vi "Message_Handler_Data.vi"(7 "Action":T5, 8 "error in (no error)":errorcluster, 9 "Time_Out":i32, 11 "Message_IN":T1={"Message Command"=enum."Process_Photo", "Parametr"={"Frame"=refnum, "Time Stamp"=timestamp(0 s since 1904-01-01), "#Frame"=0}}) -> (0 "error out":errorcluster, 1 "timed out?":bool, 3 "Message_OUT":T1={"Message Command"=enum."Process_Photo", "Parametr"={"Frame"=refnum, "Time Stamp"=timestamp(0 s since 1904-01-01), "#Frame"=0}})   [LabVIEW 2024, in "Data_Procesing.lvlib" / "Message_Handler_Data.lvlib"]
uses:
  Message_Handler_Data.lvlib
  typedeff_CommunicationModuleAction_Data.ctl
  typedeff_Message_Data.ctl
  typedeff_Message_Command_Data.ctl
  typedeff_Message_Parameters_Data.ctl
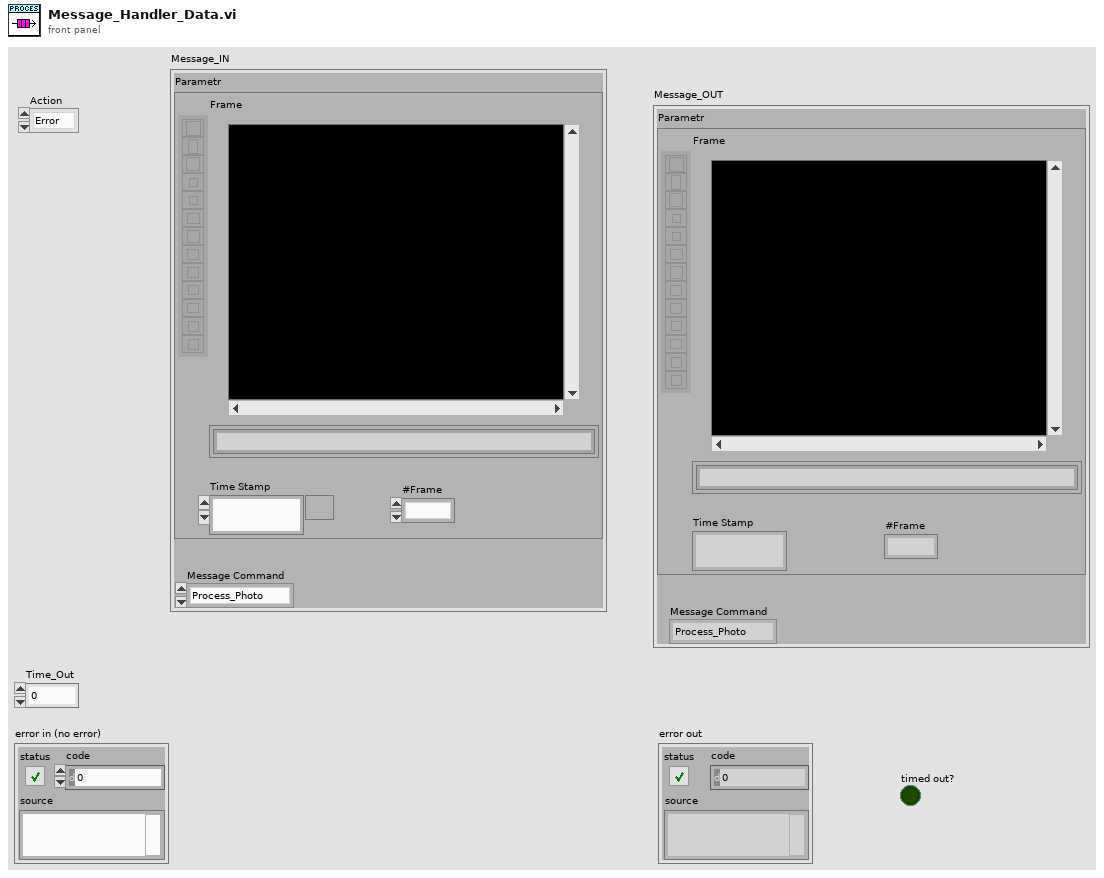
[diagram p1: front panel]
types:
  T1 = typedef "Data_Procesing.lvlib/Message_Handler_Data.lvlib/typedeff_Message_Data.ctl" = cluster{"Message Command":T2, "Parametr":T3}
  T2 = typedef "Data_Procesing.lvlib/Message_Handler_Data.lvlib/typedeff_Message_Command_Data.ctl" = enum16{"No MEssage", "Process_Photo"}
  T3 = typedef "Data_Procesing.lvlib/Message_Handler_Data.lvlib/typedeff_Message_Parameters_Data.ctl" = cluster{"Frame":T4, "Time Stamp":timestamp, "#Frame":u32}
  T4 = typedef "IMAQ Image.ctl" = refnum<image>
  T5 = typedef "Data_Procesing.lvlib/Message_Handler_Data.lvlib/typedeff_CommunicationModuleAction_Data.ctl" = enum16{"Error", "Init", "Send Msg", "Recive Msg", "Shut Down"}
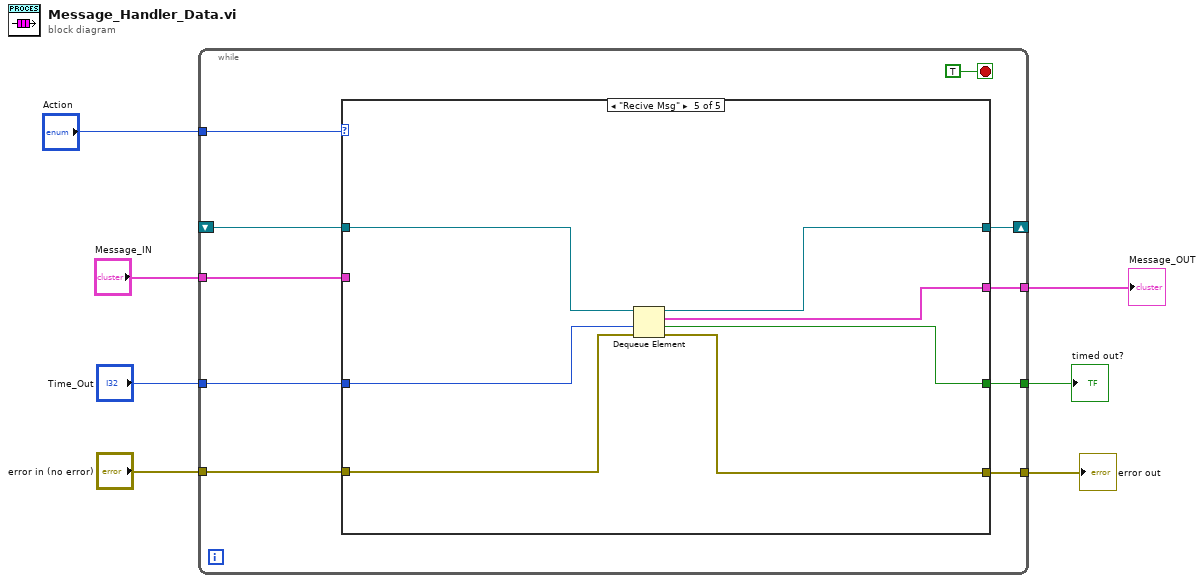
[diagram p0: block diagram]
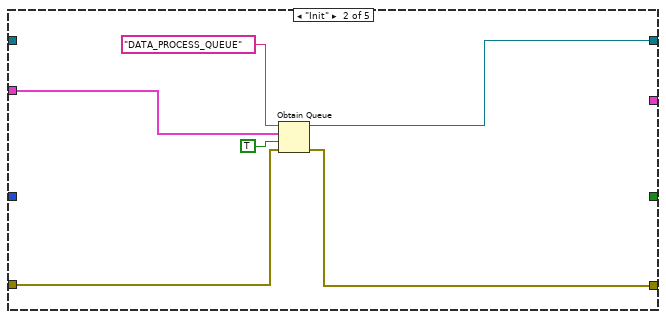
[diagram p3: hidden frame]
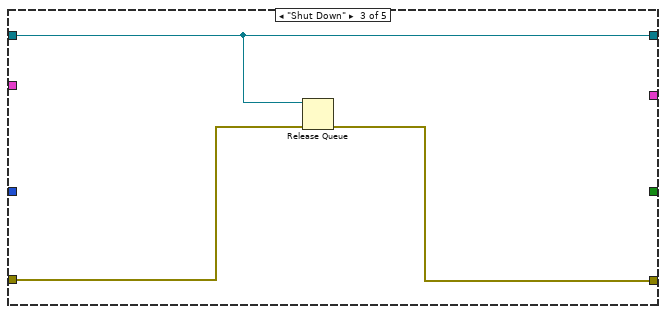
[diagram p4: hidden frame]
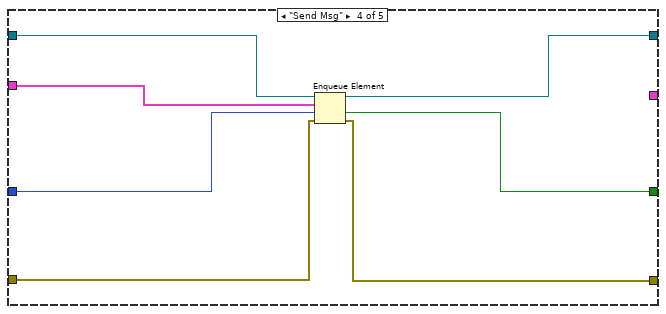
[diagram p5: hidden frame]
diagram:
  n1 = while {
    tunnel: "Action" -> [w16]
    tunnel: "error in (no error)" -> [w15]
    shift-right: [w14] -> _
    shift-left: _ -> [w13]
    tunnel: [w12] -> w6
    tunnel: "Time_Out" -> [w11]
    tunnel: [w10] -> w2
    tunnel: "Message_IN" -> [w9]
    tunnel: [w8] -> w4
    stop <- TRUE stop-if-true
    n2 = case shown="\"Recive Msg\"" w16 {
      tunnel: w15 -> [_ w23 w27 w31 w36]
      tunnel: [w18 w22 w25 w32 w39] -> w14
      tunnel: w13 -> [w18 _ w25 w34 w41]
      tunnel: [_ w21 w26 w30 w37] -> w12
      tunnel: w11 -> [_ _ _ w33 w40]
      tunnel: [_ _ _ _ w38] -> w10
      tunnel: w9 -> [_ w19 _ w29 _]
      tunnel: [_ _ _ w28 w35] -> w8
      frame "Error", Default {
      }
      frame "Init" {
        n3 = Obtain Queue(name (unnamed)="DATA_PROCESS_QUEUE", element data type=w19, create if not found? (T)=TRUE, error in (no error)=w23) -> (queue out=w22:refnum<queue>, error out=w21:errorcluster)  [unwired: 1 in, 1 out]
      }
      frame "Shut Down" {
        n4 = Release Queue(queue=w25, error in (no error)=w27) -> (error out=w26:errorcluster)  [unwired: 1 in, 2 out]
      }
      frame "Send Msg" {
        n5 = Enqueue Element(queue=w34, element=w29, timeout in ms (-1)=w33, error in (no error)=w31) -> (queue out=w32:refnum<queue>, timed out?=w28:bool, error out=w30:errorcluster)
      }
      frame "Recive Msg" {
        n6 = Dequeue Element(queue=w41, timeout in ms (-1)=w40, error in (no error)=w36) -> (queue out=w39:refnum<queue>, element=w38:T1, timed out?=w35:bool, error out=w37:errorcluster)
      }
    }
  }
  "error out" <- w6
  "timed out?" <- w4
  "Message_OUT" <- w2
